vi "AUTO - REVERSE & SHOOT.vi"(8 "error in (no error)":errorcluster) -> (0 "error out":errorcluster)   [LabVIEW 2020]
uses:
  Robot Global Data.vi
  <vilib>/Rock Robotics/Network Tables/NT Write Boolean.vi
  <vilib>/Rock Robotics/WPI/Utilities/WPI_GetSetVariantRefNum.vi
  <vilib>/Rock Robotics/Network Tables/NT Read Number.vi
  <vilib>/Rock Robotics/Network Tables/NT Write Number.vi
  <vilib>/Rock Robotics/Network Tables/NT Read Boolean.vi
panel:
  in  "KICKER refnum name":string="KICKER"
  in  "SHOOTER refname root":string="SHOOTER"
  out "SHOOTER PREV%":dbl
  in  "TURN KICKER TIME (s)":dbl=2.0 format="%#_13g"
  in  "WAIT for SHOOTER TO SPOOL UP (s)":dbl=1.5 format="%#_13g"
  in  "SHOOTER VEL %":dbl=0.65 format="%#_13g"
  in  "DRIVE TIME (s)":dbl=2.0 format="%#_13g"
  in  "DRIVE % FWD(+)":dbl=-0.5 format="%#_13g"
  out "RESET Phoenix":bool[](array[boolean])
  out "RESET SparkMAX":bool[](array[boolean])
  out "RESET Phoenix 2":bool[](array[boolean])
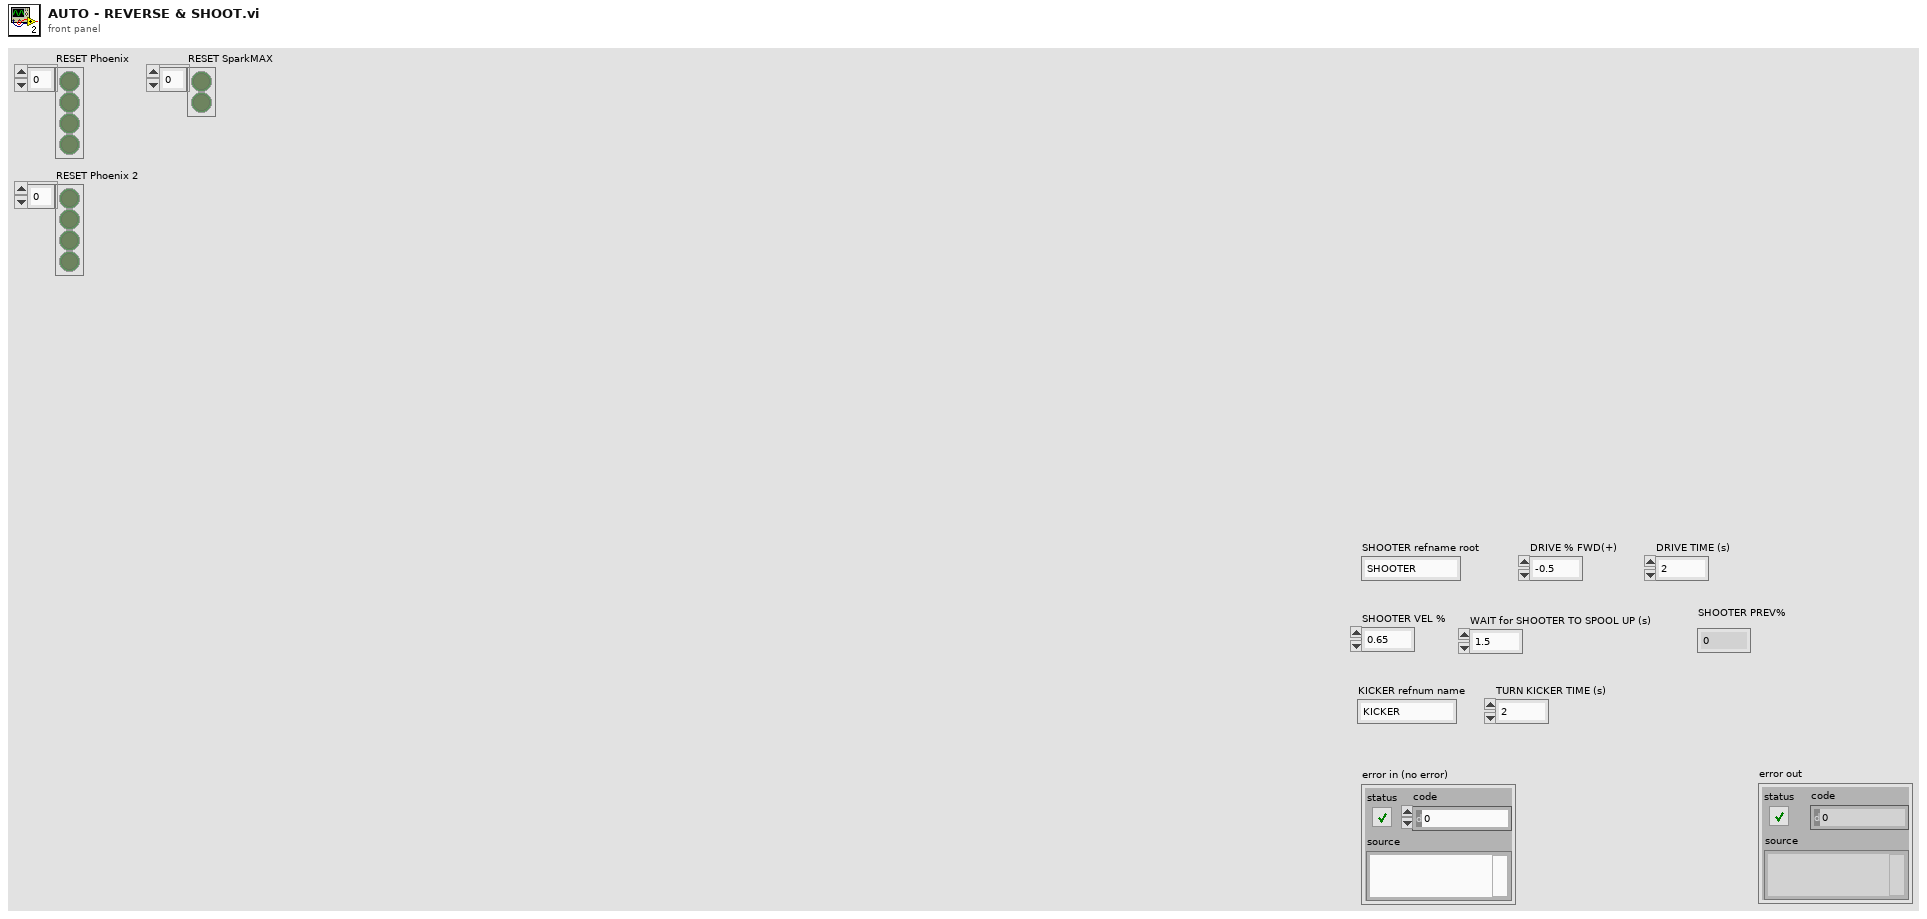
[diagram p1: front panel]
types:
  T1 = cluster{"MIN":dbl, "MAX":dbl, "convert climber inches to tics":dbl, "INITIALIZE":dbl}
  T2 = typedef "WPI_RobotDriveDevRef.ctl" = cluster{"DevStatus":errorcluster, "Motors[]":T3[], "Square Inputs":bool, "Max Output":dbl}
  T3 = typedef "WPI_MotorControlDeviceRef.ctl" = cluster{"DeviceStatus":errorcluster, "Type":T4, "PWM":cluster{"PWM Channel":T5, "DeadBand":T6}, "CAN":cluster{"Device Number":u8, "SetOutput VI Ref":variant, "GetOutput VI Ref":variant, "Enable VI Ref":variant, "Disable VI Ref":variant, "Data":variant}, "Invert":bool, "DIO PWM":cluster{"PWM \"Enable\" Channel":T5, "DIOChannel":T7, "PWM Rate":dbl}}
  T4 = typedef "WPI_MotorControlType.ctl" = enum16{"PWM", "CAN", "DIO PWM"}
  T5 = typedef "FPGA_DIOPWMChannel.ctl" = enum8{"PWM 0", "PWM 1", "PWM 2", "PWM 3", "PWM 4", "PWM 5", "PWM 6", "PWM 7", "PWM 8", "PWM 9", "PWM MXP 0", "PWM MXP 1", "PWM MXP 2", "PWM MXP 3", "PWM MXP 4", "PWM MXP 5", "PWM MXP 6", "PWM MXP 7", "PWM MXP 8", "PWM MXP 9", "Invalid"}
  T6 = typedef "WPI_PWMDeadband.ctl" = cluster{"Name":string, "maxPositivePwm":i32, "minPositivePwm":i32, "centerPwm":i32, "maxNegativePwm":i32, "minNegativePwm":i32, "angularRange":u16}
  T7 = typedef "FPGA_DIOChannel.ctl" = enum8{"DIO 0", "DIO 1", "DIO 2", "DIO 3", "DIO 4", "DIO 5", "DIO 6", "DIO 7", "DIO 8", "DIO 9", "DIO MXP 0", "DIO MXP 1", "DIO MXP 2", "DIO MXP 3", "DIO MXP 4", "DIO MXP 5", "DIO MXP 6", "DIO MXP 7", "DIO MXP 8", "DIO MXP 9", "DIO MXP 10", "DIO MXP 11", "DIO MXP 12", "DIO MXP 13", "DIO MXP 14", "DIO MXP 15", "SPI Port CS1", "SPI Port CS2", "SPI Port CS3", "SPI Port MISO", "SPI Port MOSI", "Invalid"}
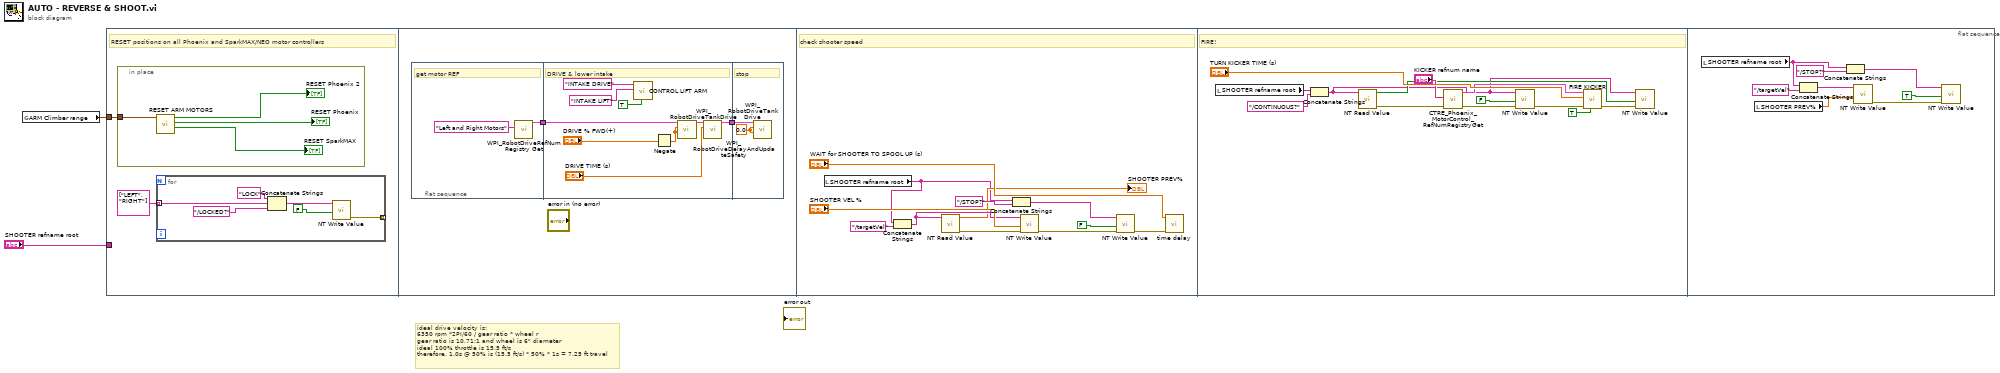
[diagram p0: block diagram]
diagram:
  # "ideal drive velocity is:\n6350 rpm *2PI/60 / gear ratio * wheel r\ngear ratio is 10.71:1 and wheel is 6\" diameter\nideal 100% throttle is 15.5 ft/s\ntherefore, 1.0s @ 50% is (15.5 ft/s) * 50% * 1s = 7.25 ft travel"
  n1 = global read "Robot Global Data.vi" "ARM Climber range"() -> (w2:T1)
  n2 = flat-sequence {
    tunnel: w2 -> [w4]
    tunnel: "SHOOTER refname root" -> [_]
    frame #0 {
      # "RESET positions on all Phoenix and SparkMAX/NEO motor controllers"
      n3 = in-place {
        in-place-border: w4 -> [w8]
        n4 = call "RESET ARM MOTORS.vi"("ARM Climber range"=w8) -> ("RESET SparkMAX"=→"RESET SparkMAX":bool[], "RESET Phoenix"=→"RESET Phoenix":bool[], "RESET Phoenix 2"=→"RESET Phoenix 2":bool[])  [unwired: 8 in]
      }
      n5 = for {
        tunnel: string[] ["LEFT", "RIGHT"] -> [w11] mode=indexing
        tunnel: [w9] -> _ mode=indexing
        n6 = Concatenate Strings("LOCK" ("string"), w11, "/LOCKED?" ("Name")) -> (w13:string)
        n7 = call-poly <vilib>:"NT Write Value.vi"("Boolean"=FALSE, "Name"=w13) -> ("error out"=w9:errorcluster)  [unwired: 9 in]
      }
    }
    frame #1 {
      n8 = flat-sequence {
        tunnel: [w17] -> w16
        tunnel: w16 -> [w26]
        tunnel: [w25] -> w15
        tunnel: w15 -> [w29]
        frame #0 {
          # "get motor REF"
          n9 = call <vilib>:"WPI_RobotDriveRefNum Registry Get.vi"("refnum name"="Left and Right Motors") -> ("RobotDriveDevRef"=w17:T2)  [unwired: 1 in, 9 out]
        }
        frame #1 {
          # "DRIVE & lower intake"
          n10 = call "CONTROL LIFT ARM.vi"("force extend?"=TRUE, "LIFT ARM refname"="INTAKE LIFT", "LIFT DRIVE refname"="INTAKE DRIVE") -> ()  [unwired: 8 in, 1 out]
          n11 = Negate(x="DRIVE % FWD(+)") -> (-x=w19:dbl)
          n12 = call <vilib>:"WPI_RobotDriveTankDrive.vi"("Right axis value"=w19, "Left axis value"=w19, "RobotDriveDevRef"=w26) -> ("RobotDriveDevRef"=w27:T2)  [unwired: 6 in, 2 out]
          n13 = call <vilib>:"WPI_RobotDriveDelayAndUpdateSafety.vi"("Delay (s)"="DRIVE TIME (s)", "RobotDriveDevRef"=w27) -> ("RobotDriveDevRef 2"=w25:T2)  [unwired: 8 in, 1 out]
        }
        frame #2 {
          w28 = 0.0 ("X axis value")
          # "stop"
          n14 = call <vilib>:"WPI_RobotDriveTankDrive.vi"("Right axis value"=w28, "Left axis value"=w28, "RobotDriveDevRef"=w29) -> ()  [unwired: 6 in, 3 out]
        }
      }
    }
    frame #2 {
      # "check shooter speed"
      n15 = local read "SHOOTER refname root"() -> (w30:string)
      n16 = Concatenate Strings(w30, "/targetVel" ("Name")) -> (w32:string)
      n17 = call-poly <vilib>:"NT Read Value.vi"("Name"=w32) -> ("error out"=w33:errorcluster, "Numeric"=→"SHOOTER PREV%":dbl)  [unwired: 9 in]
      n18 = Concatenate Strings(w30, "/STOP?" ("string")) -> (w40:string)
      n19 = call-poly <vilib>:"NT Write Value.vi"("error in"=w33, "Numeric"="SHOOTER VEL %", "Name"=w32) -> ("error out"=w37:errorcluster)  [unwired: 8 in]
      n20 = call-poly <vilib>:"NT Write Value.vi"("error in"=w37, "Boolean"=FALSE, "Name"=w40) -> ("error out"=w36:errorcluster)  [unwired: 8 in]
      n21 = call "time delay.vi"("error in (no error)"=w36, "timer delay (s)"="WAIT for SHOOTER TO SPOOL UP (s)") -> ()  [unwired: 8 in, 2 out]
    }
    frame #3 {
      # "FIRE!"
      n22 = local read "SHOOTER refname root"() -> (w42:string)
      n23 = Concatenate Strings(w42, "/CONTINUOUS?" ("Name")) -> (w43:string)
      n24 = call-poly <vilib>:"NT Read Value.vi"("Name"=w43) -> ("error out"=w47:errorcluster, "Boolean"=w45:bool)  [unwired: 9 in]
      n25 = call <vilib>:"CTRE_Phoenix_MotorControl_RefNumRegistryGet.vi"("error in (no error)"=w47, "refnum name"="KICKER refnum name") -> ("error out"=w48:errorcluster, "PhoenixMotorControlDevRef"=w49:T3)  [unwired: 8 in]
      n26 = call-poly <vilib>:"NT Write Value.vi"("error in"=w48, "Boolean"=FALSE, "Name"=w43) -> ("error out"=w51:errorcluster)  [unwired: 8 in]
      n27 = call "FIRE KICKER.vi"("force fire?"=TRUE, "error in (no error)"=w51, "delay seconds"="TURN KICKER TIME (s)", "VictorSPX devref in"=w49) -> ("error out"=w46:errorcluster)  [unwired: 6 in, 1 out]
      n28 = call-poly <vilib>:"NT Write Value.vi"("error in"=w46, "Boolean"=w45, "Name"=w43) -> ()  [unwired: 8 in, 1 out]
    }
    frame #4 {
      n29 = local read "SHOOTER refname root"() -> (w55:string)
      n30 = local read "SHOOTER PREV%"() -> (w56:dbl)
      n31 = Concatenate Strings(w55, "/targetVel" ("Name")) -> (w62:string)
      n32 = Concatenate Strings(w55, "/STOP?" ("string")) -> (w60:string)
      n33 = call-poly <vilib>:"NT Write Value.vi"("Numeric"=w56, "Name"=w62) -> ("error out"=w57:errorcluster)  [unwired: 9 in]
      n34 = call-poly <vilib>:"NT Write Value.vi"("error in"=w57, "Boolean"=TRUE, "Name"=w60) -> ()  [unwired: 8 in, 1 out]
    }
  }
